vi "GSP_MasterConfiguration.vi"(5 "error in (no error)":errorcluster, 6 "Slit File":path, 7 "Filter File":path, 8 "grating file":path) -> (0 "error out":errorcluster, 2 "Changes Made?":bool)   [LabVIEW 2015]
uses:
  Misc/GUI_Buttons_23x22_W2K.llb/ArrowLeftBlue.ctl
  Misc/GUI_Buttons_23x22_W2K.llb/Delete1.ctl
  Dialog/dialog_messages.ctl
  GSP_GUI_global.vi
panel:
  in  "Clear Changes":bool
  in  "Load from Config":bool
  in  "Apply Changes":bool
  in  "Tab Control":T1(tab)=enum."Slit Carousel"
  in  "5-hole (SQUARE)":bool caption="6-hole (ROUND)"
  out "Filter Info":string
  in  "Remove Secondary":T2
  in  "Load Secondary":T3
  in  "Remove Primary":T2
  in  "Load Primary":T3
  in  "Available Filters":i32(listbox)
  in  "Secondary Filter Wheel Listbox":i32(listbox) caption="Secondary"
  in  "Primary Filter Wheel Listbox":i32(listbox) caption="Primary"
  out "Grating Info":string
  in  "Available Gratings":i32(listbox)
  in  "Remove  Grating":T2
  in  "Load Grating":T3
  in  "Grating Tray Listbox":i32(listbox)
  out "Slit Info":string
  in  "Available Slits":i32(listbox)
  in  "Remove  Slit":T2
  in  "Load Slit":T3
  in  "Slit Mask Listbox":i32(listbox)
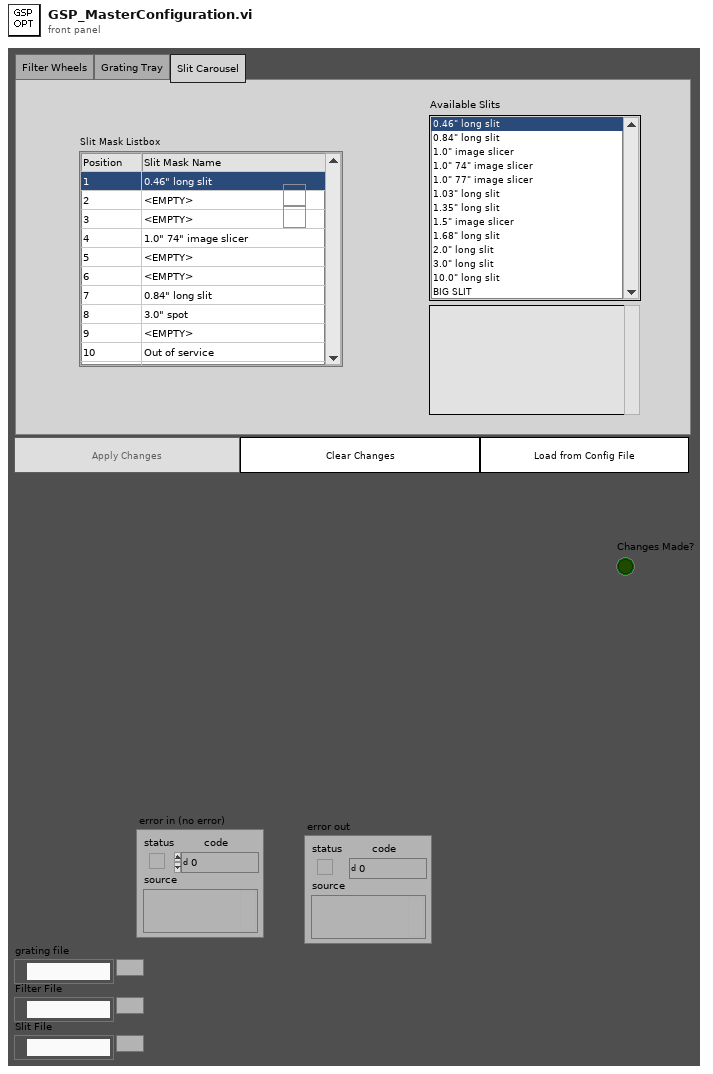
[diagram p1: front panel]
types:
  T1 = enum32{"Filter Wheels", "Grating Tray", "Slit Carousel"}
  T2 = typedef "Delete1.ctl" = bool
  T3 = typedef "ArrowLeftBlue.ctl" = bool
  T4 = typedef "dialog_messages.ctl" = enum16{"Custom", "Incompatible Config"}
  T5 = cluster{"Primary Filter Names":string[], "Secondary Filter Names":string[], "Grating Names":string[], "Slit Mask Names":string[]}
  T6 = cluster{"Comment":string, "lines/mm":i32, "modulation":dbl, "thickness (mm)":dbl}
  T7 = cluster{"Comment":string, "Width":dbl, "Observer":string, "Field":string}
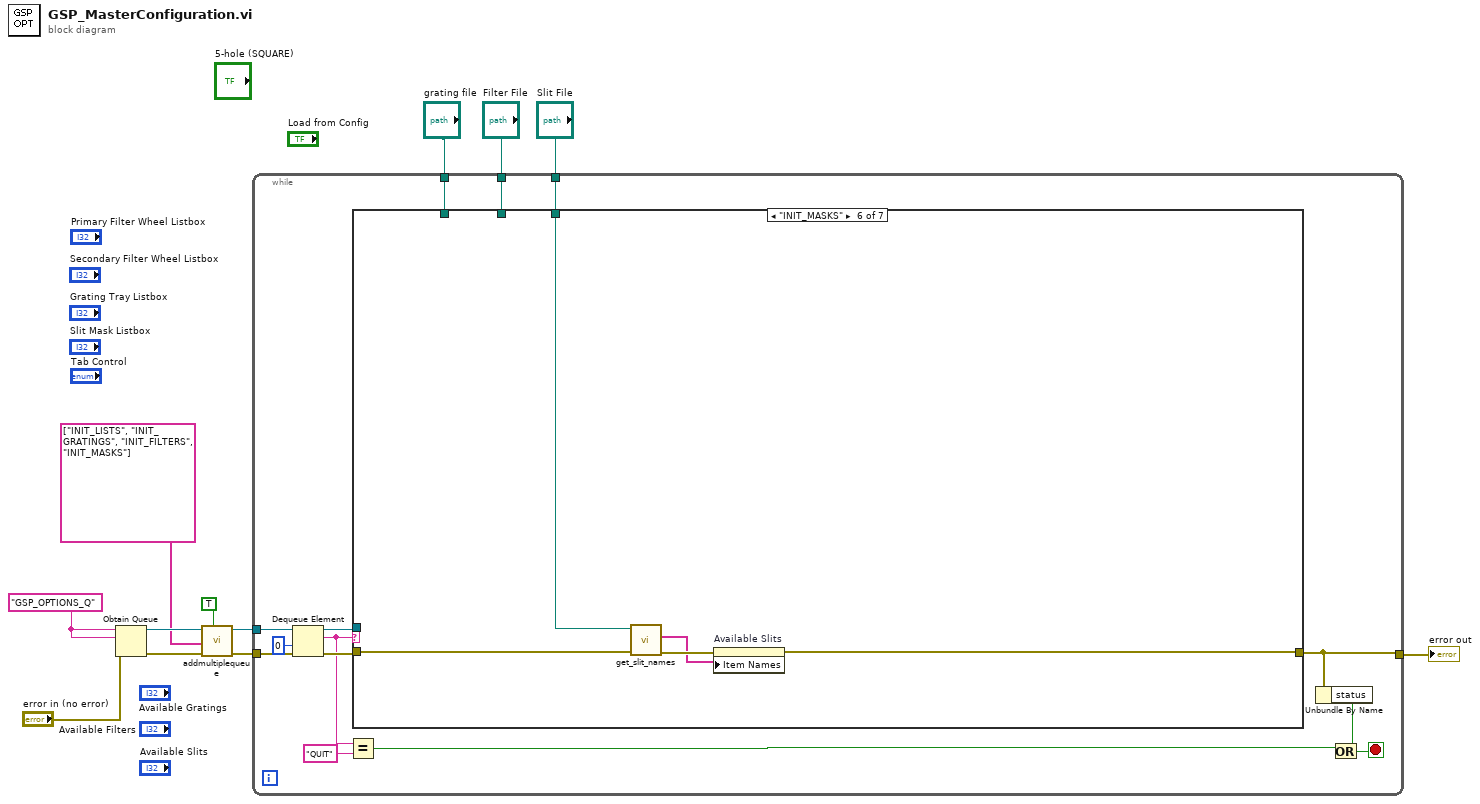
[diagram p0: block diagram]
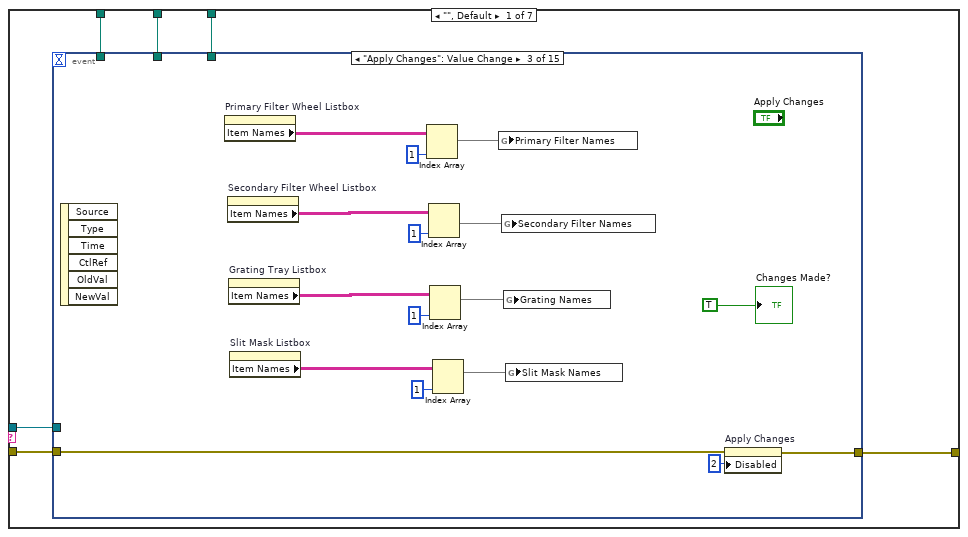
[diagram p2: hidden frame]
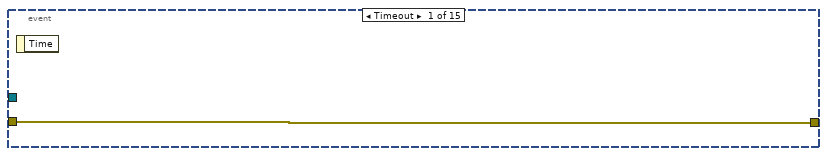
[diagram p3: hidden frame]
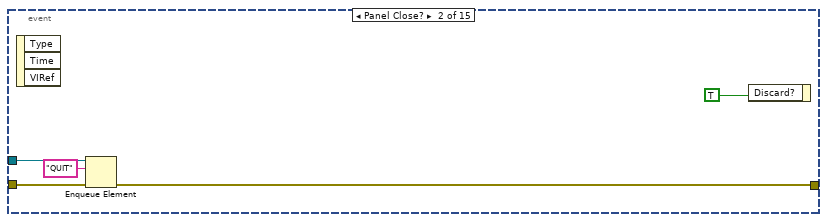
[diagram p4: hidden frame]
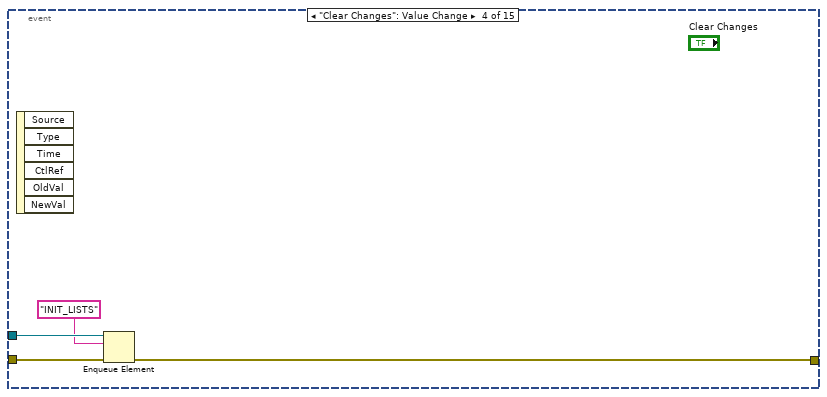
[diagram p5: hidden frame]
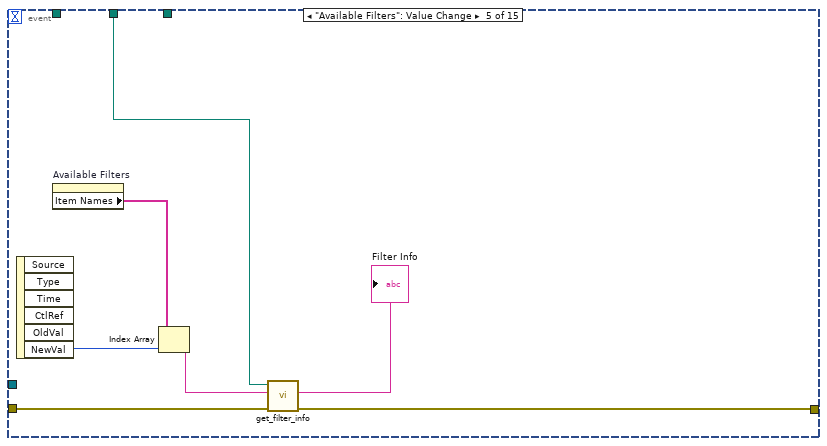
[diagram p6: hidden frame]
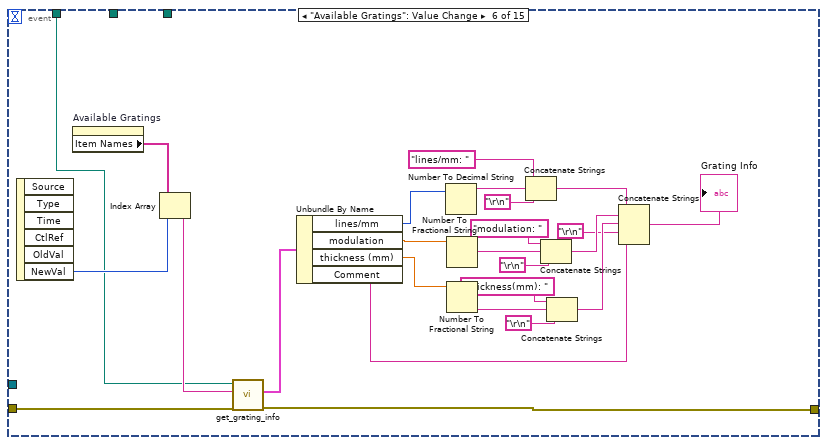
[diagram p7: hidden frame]
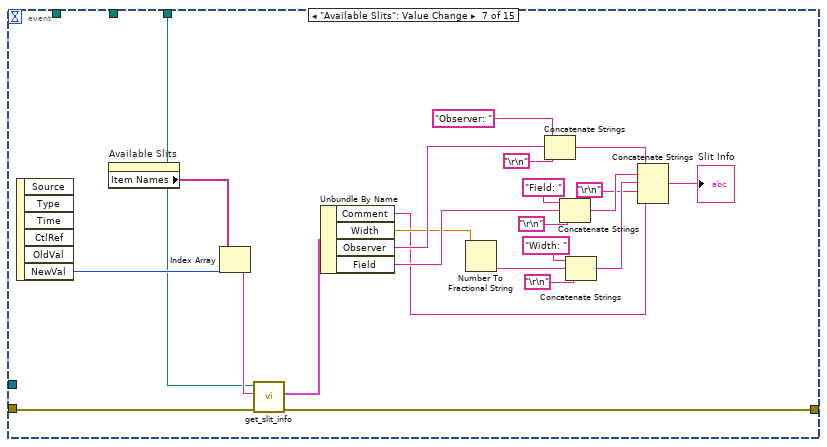
[diagram p8: hidden frame]
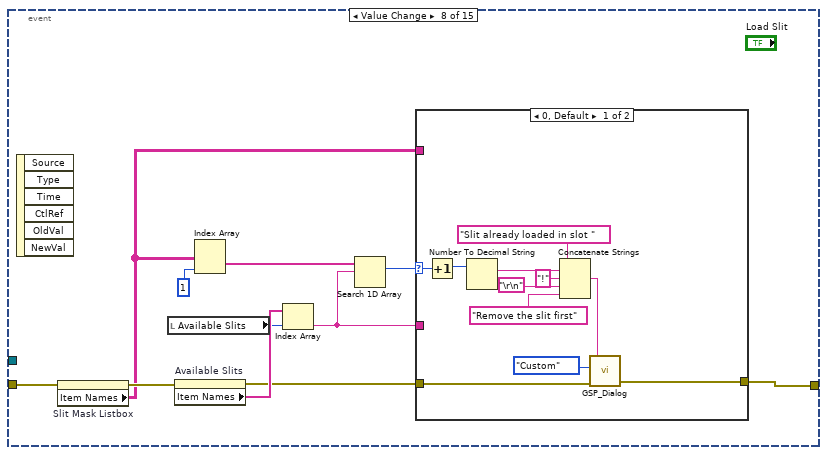
[diagram p9: hidden frame]
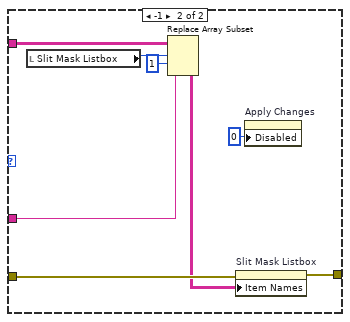
[diagram p10: hidden frame]
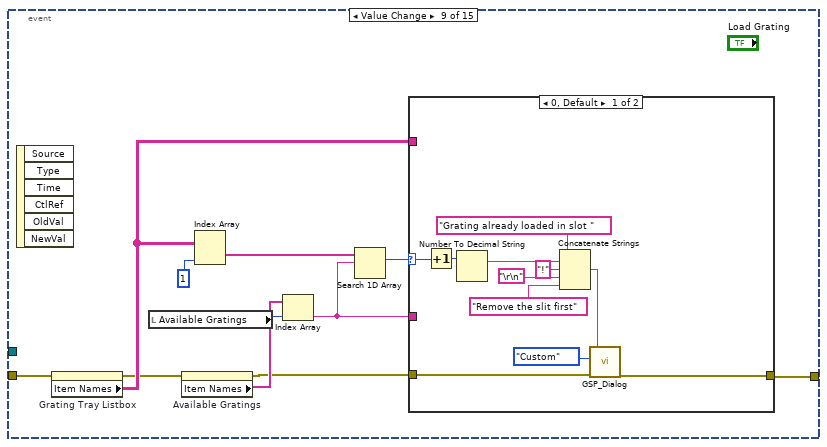
[diagram p11: hidden frame]
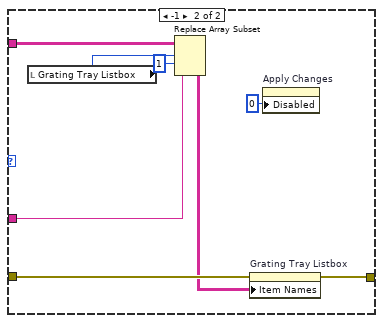
[diagram p12: hidden frame]
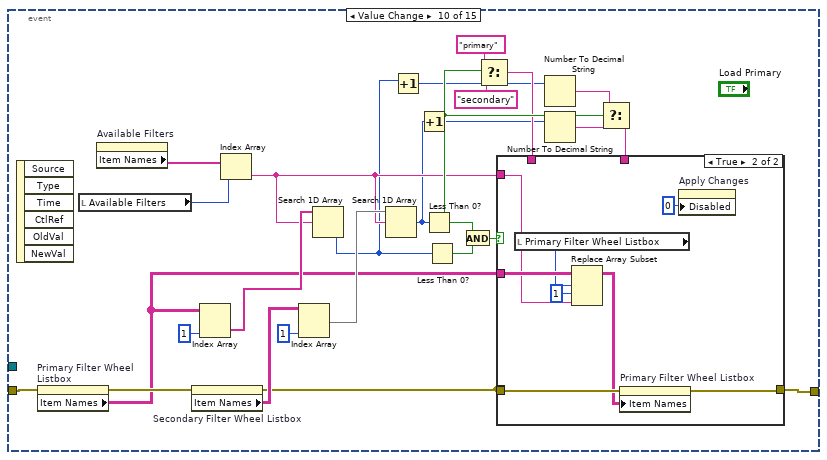
[diagram p13: hidden frame]
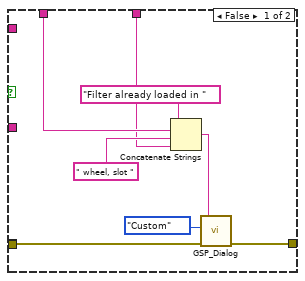
[diagram p14: hidden frame]
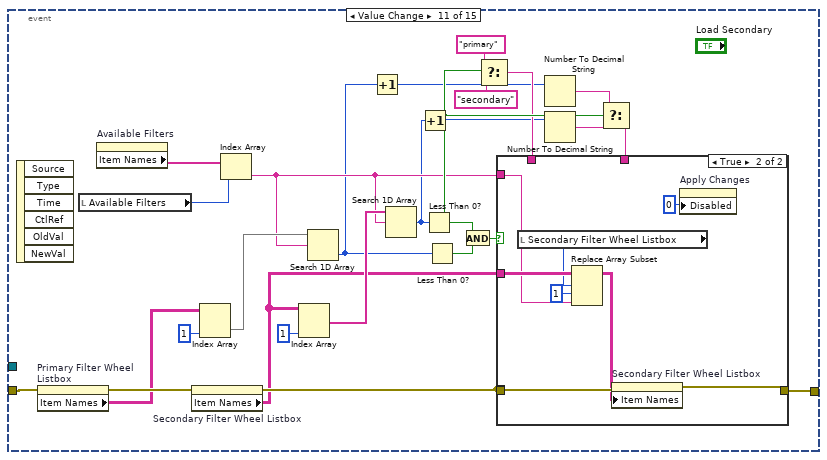
[diagram p15: hidden frame]
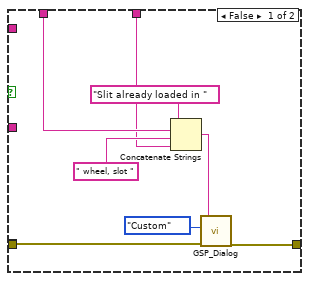
[diagram p16: hidden frame]
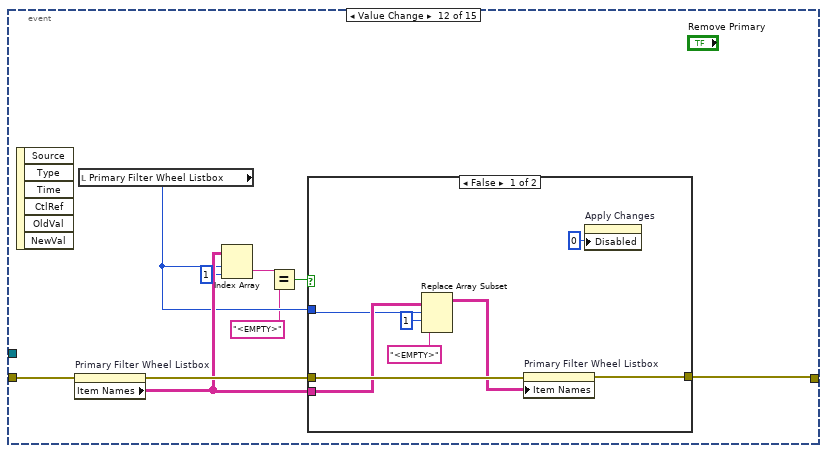
[diagram p17: hidden frame]
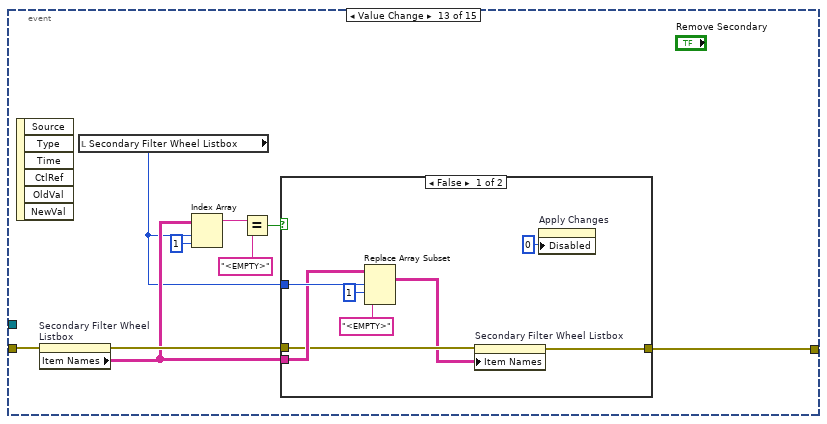
[diagram p19: hidden frame]
diagram:
  w12 = "GSP_OPTIONS_Q" ("name (unnamed)")
  n1 = Obtain Queue(name (unnamed)=w12, element data type=w12, error in (no error)="error in (no error)") -> (queue out=w11:refnum<queue>, error out=w10:errorcluster)  [unwired: 2 in, 1 out]
  n2 = call "addmultiplequeue.vi"("Add All (false)"=TRUE, "error in (no error)"=w10, "Strings to Add"=string[] ["INIT_LISTS", "INIT_GRATINGS", "INIT_FILTERS", "INIT_MASKS"], "queue"=w11) -> ("error out"=w9:errorcluster, "queue out"=w8:refnum<queue>)  [unwired: 3 in]
  n3 = while {
    tunnel: w9 -> [w25]
    tunnel: w8 -> [w26]
    tunnel: [w16] -> w6
    tunnel: "grating file" -> [w15]
    tunnel: "Filter File" -> [w14]
    tunnel: "Slit File" -> [w13]
    stop <- w19 stop-if-true
    n4 = Dequeue Element(queue=w26, timeout in ms (-1)=0, error in (no error)=w25) -> (queue out=w23:refnum<queue>, element=w21:string, error out=w22:errorcluster)  [unwired: 1 out]
    n5 = Equal?(x=w21, y="QUIT") -> (x = y?=w18:bool)
    n6 = case shown="\"INIT_MASKS\"" w21 {
      tunnel: w23 -> [w31 _ _ _ _ _ _]
      tunnel: w22 -> [w32 w345 w360 w384 w391 w396 w397]
      tunnel: [w30 w339 w360 w386 w388 w393 w397] -> w16
      tunnel: w15 -> [w28 _ _ w382 _ _ _]
      tunnel: w14 -> [w29 _ _ _ w387 _ _]
      tunnel: w13 -> [w27 _ _ _ _ w392 _]
      frame "", Default {
        n7 = event shown="[2] \"Apply Changes\": Value Change" {
          selector: _ -> [_ _ _ _ _ _ _ _ _ _ _ _ _ _ _]
          dyn-events: _ -> [_ _ _ _ _ _ _ _ _ _ _ _ _ _ _]
          timeout: _ -> [_ _ _ _ _ _ _ _ _ _ _ _ _ _ _]
          tunnel: w32 -> [w33 w36 w43 w57 w63 w68 w101 w124 w149 w199 w241 w266 w284 w302 w320]
          tunnel: w31 -> [_ w37 _ w58 _ _ _ _ _ _ _ _ _ _ _]
          tunnel: [w33 w35 w44 w56 w60 w69 w99 w117 w152 w188 w231 w264 w282 w300 w318] -> w30
          tunnel: w29 -> [_ _ _ _ w59 _ _ _ _ _ _ _ _ _ _]
          tunnel: w28 -> [_ _ _ _ _ w66 _ _ _ _ _ _ _ _ _]
          tunnel: w27 -> [_ _ _ _ _ _ w91 _ _ _ _ _ _ _ _]
          event Timeout {
            n8 = event-data() -> ()  [unwired: 1 in, 1 out]
          }
          event Panel Close? {
            n9 = event-data() -> ()  [unwired: 1 in, 3 out]
            n10 = Enqueue Element(queue=w37, element="QUIT", error in (no error)=w36) -> (error out=w35:errorcluster)  [unwired: 1 in, 2 out]
            n11 = event-data("Discard?"=TRUE) -> ()  [unwired: 1 in, 1 out]
          }
          event "Apply Changes": Value Change {
            n12 = event-data() -> ()  [unwired: 1 in, 6 out]
            n13 = property on="Primary Filter Wheel Listbox" class="MCListbox (strict)"() -> ("Item Names"=w53:string[][])  [unwired: 2 in, 2 out]
            n14 = property on="Secondary Filter Wheel Listbox" class="MCListbox (strict)"() -> ("Item Names"=w48:string[][])  [unwired: 2 in, 2 out]
            n15 = property on="Grating Tray Listbox" class="MCListbox (strict)"() -> ("Item Names"=w47:string[][])  [unwired: 2 in, 2 out]
            n16 = property on="Slit Mask Listbox" class="MCListbox (strict)"() -> ("Item Names"=w46:string[][])  [unwired: 2 in, 2 out]
            n17 = Index Array(array=w53, index (col)=1 ("disabled index (col)")) -> (element=w39:string[])  [unwired: 1 in]
            n18 = Index Array(array=w48, index (col)=1 ("disabled index (col)")) -> (element=w40:string[])  [unwired: 1 in]
            n19 = Index Array(array=w47, index (col)=1 ("disabled index (col)")) -> (element=w41:string[])  [unwired: 1 in]
            n20 = Index Array(array=w46, index (col)=1 ("disabled index (col)")) -> (element=w42:string[])  [unwired: 1 in]
            n21 = global write "GSP_GUI_global.vi" "Primary Filter Names"(w39) -> ()
            n22 = global write "GSP_GUI_global.vi" "Secondary Filter Names"(w40) -> ()
            n23 = global write "GSP_GUI_global.vi" "Grating Names"(w41) -> ()
            n24 = global write "GSP_GUI_global.vi" "Slit Mask Names"(w42) -> ()
            n25 = property on="Apply Changes" class="Bool"(error in=w43, "Disabled"=u8 2) -> (error out=w44:errorcluster)  [unwired: 1 in, 1 out]
            "Changes Made?" <- TRUE
          }
          event "Clear Changes": Value Change {
            n26 = event-data() -> ()  [unwired: 1 in, 6 out]
            n27 = Enqueue Element(queue=w58, element="INIT_LISTS", error in (no error)=w57) -> (error out=w56:errorcluster)  [unwired: 1 in, 2 out]
          }
          event "Available Filters": Value Change {
            n28 = event-data() -> ("NewVal"=w65:i32)  [unwired: 1 in, 5 out]
            n29 = property on="Available Filters" class="LstBox (strict)"() -> ("Item Names"=w64:string[])  [unwired: 2 in, 2 out]
            n30 = Index Array(array=w64, index=w65) -> (element=w62:string)
            n31 = call "get_filter_info.vi"("error in (no error)"=w63, "filter name"=w62, "configuration file path"=w59) -> ("error out"=w60:errorcluster, "Comment"=→"Filter Info":string)  [unwired: 3 in]
          }
          event "Available Gratings": Value Change {
            n32 = event-data() -> ("NewVal"=w90:i32)  [unwired: 1 in, 5 out]
            n33 = property on="Available Gratings" class="LstBox (strict)"() -> ("Item Names"=w89:string[])  [unwired: 2 in, 2 out]
            n34 = Index Array(array=w89, index=w90) -> (element=w67:string)
            n35 = call "get_grating_info.vi"("error in (no error)"=w68, "grating name"=w67, "configuration file path"=w66) -> ("error out"=w69:errorcluster, "Grating Info"=w70:T6)  [unwired: 3 in]
            n36 = Unbundle By Name(w70) -> ("lines/mm"=w88:i32, "modulation"=w87:dbl, "thickness (mm)"=w86:dbl, "Comment"=w73:string)
            n37 = Number To Decimal String(number=w88) -> (decimal integer string=w85:string)  [unwired: 1 in]
            n38 = Number To Fractional String(number=w87) -> (F-format string=w81:string)  [unwired: 3 in]
            n39 = Number To Fractional String(number=w86) -> (F-format string=w71:string)  [unwired: 3 in]
            n40 = Concatenate Strings("lines/mm: ", w85, "\r\n") -> (w77:string)
            n41 = Concatenate Strings("modulation: " ("string"), w81, "\r\n") -> (w76:string)
            n42 = Concatenate Strings("thickness(mm): " ("string"), w71, "\r\n") -> (w75:string)
            n43 = Concatenate Strings(w77, w76, w75, "\r\n", w73) -> (→"Grating Info":string)
          }
          event "Available Slits": Value Change {
            n44 = event-data() -> ("NewVal"=w113:i32)  [unwired: 1 in, 5 out]
            n45 = property on="Available Slits" class="LstBox (strict)"() -> ("Item Names"=w112:string[])  [unwired: 2 in, 2 out]
            n46 = Index Array(array=w112, index=w113) -> (element=w100:string)
            n47 = call "get_slit_info.vi"("error in (no error)"=w101, "mask name"=w100, "configuration file path"=w91) -> ("error out"=w99:errorcluster, "Slit Info"=w98:T7)  [unwired: 3 in]
            n48 = Unbundle By Name(w98) -> ("Comment"=w93:string, "Width"=w95:dbl, "Observer"=w97:string, "Field"=w96:string)
            n49 = Number To Fractional String(number=w95) -> (F-format string=w102:string)  [unwired: 3 in]
            n50 = Concatenate Strings("Observer: ", w97, "\r\n") -> (w94:string)
            n51 = Concatenate Strings("Field: " ("string"), w96, "\r\n") -> (w105:string)
            n52 = Concatenate Strings("Width: " ("string"), w102, "\r\n") -> (w104:string)
            n53 = Concatenate Strings(w94, w105, w104, "\r\n", w93) -> (→"Slit Info":string)
          }
          event Value Change {
            n54 = event-data() -> ()  [unwired: 1 in, 6 out]
            n55 = property on="Slit Mask Listbox" class="MCListbox (strict)"(error in=w124) -> (error out=w123:errorcluster, "Item Names"=w115:string[][])  [unwired: 1 in, 1 out]
            n56 = local read "Available Slits"() -> (w121:i32)
            n57 = property on="Available Slits" class="LstBox (strict)"(error in=w123) -> (error out=w118:errorcluster, "Item Names"=w122:string[])  [unwired: 1 in, 1 out]
            n58 = Index Array(array=w115, index (col)=1 ("disabled index (col)")) -> (element=w116:string[])  [unwired: 1 in]
            n59 = Index Array(array=w122, index=w121) -> (element=w114:string)
            n60 = Search 1D Array(1D array=w116, element=w114) -> (index of element=w119:i32)  [unwired: 1 in]
            n61 = case shown="0, Default" w119 {
              selector: w119 -> [w126 _]
              tunnel: w118 -> [w134 w143]
              tunnel: [w133 w142] -> w117
              tunnel: w115 -> [_ w141]
              tunnel: w114 -> [_ w138]
              frame 0, Default {
                n62 = Increment(x=w126) -> (x+1=w125:i32)
                n63 = Number To Decimal String(number=w125) -> (decimal integer string=w132:string)  [unwired: 1 in]
                n64 = Concatenate Strings("Slit already loaded in slot " ("Message"), w132, "!" ("string"), "\r\n", "Remove the slit first" ("string")) -> (w130:string)
                n65 = call "GSP_Dialog.vi"("error in (no error)"=w134, "Messages"=dialog_messages."Custom", "Message"=w130) -> ("error out"=w133:errorcluster)  [unwired: 4 in]
              }
              frame -1 {
                n66 = local read "Slit Mask Listbox"() -> (w139:i32)
                n67 = Replace Array Subset(array=w141, new element=w138, index (row)=w139, index (col)=1 ("disabled index (col)")) -> (w137:string[][])
                n68 = property on="Slit Mask Listbox" class="MCListbox (strict)"(error in=w143, "Item Names"=w137) -> (error out=w142:errorcluster)  [unwired: 1 in, 1 out]
                n69 = property on="Apply Changes" class="Bool"("Disabled"=u8 0) -> ()  [unwired: 2 in, 2 out]
              }
            }
          }
          event Value Change {
            n70 = event-data() -> ()  [unwired: 1 in, 6 out]
            n71 = property on="Grating Tray Listbox" class="MCListbox (strict)"(error in=w149) -> (error out=w147:errorcluster, "Item Names"=w148:string[][])  [unwired: 1 in, 1 out]
            n72 = local read "Available Gratings"() -> (w144:i32)
            n73 = property on="Available Gratings" class="LstBox (strict)"(error in=w147) -> (error out=w145:errorcluster, "Item Names"=w146:string[])  [unwired: 1 in, 1 out]
            n74 = Index Array(array=w148, index (col)=1 ("disabled index (col)")) -> (element=w151:string[])  [unwired: 1 in]
            n75 = Index Array(array=w146, index=w144) -> (element=w150:string)
            n76 = Search 1D Array(1D array=w151, element=w150) -> (index of element=w153:i32)  [unwired: 1 in]
            n77 = case shown="0, Default" w153 {
              selector: w153 -> [w156 _]
              tunnel: w145 -> [w164 w169]
              tunnel: [w163 w168] -> w152
              tunnel: w148 -> [_ w173]
              tunnel: w150 -> [_ w171]
              frame 0, Default {
                n78 = Increment(x=w156) -> (x+1=w155:i32)
                n79 = Number To Decimal String(number=w155) -> (decimal integer string=w162:string)  [unwired: 1 in]
                n80 = Concatenate Strings("Grating already loaded in slot " ("Message"), w162, "!" ("string"), "\r\n", "Remove the slit first" ("string")) -> (w160:string)
                n81 = call "GSP_Dialog.vi"("error in (no error)"=w164, "Messages"=dialog_messages."Custom", "Message"=w160) -> ("error out"=w163:errorcluster)  [unwired: 4 in]
              }
              frame -1 {
                n82 = local read "Grating Tray Listbox"() -> (w170:i32)
                n83 = Replace Array Subset(array=w173, new element=w171, index (row)=w170, index (col)=1 ("disabled index (col)")) -> (w167:string[][])
                n84 = property on="Grating Tray Listbox" class="MCListbox (strict)"(error in=w169, "Item Names"=w167) -> (error out=w168:errorcluster)  [unwired: 1 in, 1 out]
                n85 = property on="Apply Changes" class="Bool"("Disabled"=u8 0) -> ()  [unwired: 2 in, 2 out]
              }
            }
          }
          event Value Change {
            n86 = event-data() -> ()  [unwired: 1 in, 6 out]
            n87 = property on="Primary Filter Wheel Listbox" class="MCListbox (strict)"(error in=w199) -> (error out=w198:errorcluster, "Item Names"=w178:string[][])  [unwired: 1 in, 1 out]
            n88 = local read "Available Filters"() -> (w196:i32)
            n89 = property on="Available Filters" class="LstBox (strict)"() -> ("Item Names"=w197:string[])  [unwired: 2 in, 2 out]
            n90 = property on="Secondary Filter Wheel Listbox" class="MCListbox (strict)"(error in=w198) -> (error out=w179:errorcluster, "Item Names"=w193:string[][])  [unwired: 1 in, 1 out]
            n91 = Index Array(array=w178, index (col)=1 ("disabled index (col)")) -> (element=w192:string[])  [unwired: 1 in]
            n92 = Index Array(array=w197, index=w196) -> (element=w180:string)
            n93 = Index Array(array=w193, index (col)=1 ("disabled index (col)")) -> (element=w191:string[])  [unwired: 1 in]
            n94 = Search 1D Array(1D array=w192, element=w180) -> (index of element=w177:i32)  [unwired: 1 in]
            n95 = Search 1D Array(1D array=w191, element=w180) -> (index of element=w175:i32)  [unwired: 1 in]
            n96 = Increment(x=w177) -> (x+1=w176:i32)
            n97 = Increment(x=w175) -> (x+1=w174:i32)
            n98 = Less Than 0?(x=w175) -> (x < 0?=w183:bool)
            n99 = Less Than 0?(x=w177) -> (x < 0?=w190:bool)
            n100 = And(x=w183, y=w190) -> (x .and. y?=w189:bool)
            n101 = Select(t="primary", s=w183, f="secondary") -> (s? t:f=w182:string)
            n102 = Number To Decimal String(number=w176) -> (decimal integer string=w185:string)  [unwired: 1 in]
            n103 = Number To Decimal String(number=w174) -> (decimal integer string=w184:string)  [unwired: 1 in]
            n104 = Select(t=w185, s=w183, f=w184) -> (s? t:f=w181:string)
            n105 = case shown="True" w189 {
              tunnel: w179 -> [w205 _]
              tunnel: [w204 w214] -> w188
              tunnel: w182 -> [w202 _]
              tunnel: w181 -> [w200 _]
              tunnel: w180 -> [_ w210]
              tunnel: w179 -> [_ w215]
              tunnel: w178 -> [_ w213]
              frame False {
                n106 = Concatenate Strings("Filter already loaded in " ("Message"), w202, " wheel, slot ", w200) -> (w206:string)
                n107 = call "GSP_Dialog.vi"("error in (no error)"=w205, "Messages"=dialog_messages."Custom", "Message"=w206) -> ("error out"=w204:errorcluster)  [unwired: 4 in]
              }
              frame True {
                n108 = local read "Primary Filter Wheel Listbox"() -> (w211:i32)
                n109 = Replace Array Subset(array=w213, new element=w210, index (row)=w211, index (col)=1 ("disabled index (col)")) -> (w209:string[][])
                n110 = property on="Primary Filter Wheel Listbox" class="MCListbox (strict)"(error in=w215, "Item Names"=w209) -> (error out=w214:errorcluster)  [unwired: 1 in, 1 out]
                n111 = property on="Apply Changes" class="Bool"("Disabled"=u8 0) -> ()  [unwired: 2 in, 2 out]
              }
            }
          }
          event Value Change {
            n112 = event-data() -> ()  [unwired: 1 in, 6 out]
            n113 = property on="Primary Filter Wheel Listbox" class="MCListbox (strict)"(error in=w241) -> (error out=w240:errorcluster, "Item Names"=w223:string[][])  [unwired: 1 in, 1 out]
            n114 = local read "Available Filters"() -> (w238:i32)
            n115 = property on="Available Filters" class="LstBox (strict)"() -> ("Item Names"=w239:string[])  [unwired: 2 in, 2 out]
            n116 = property on="Secondary Filter Wheel Listbox" class="MCListbox (strict)"(error in=w240) -> (error out=w224:errorcluster, "Item Names"=w222:string[][])  [unwired: 1 in, 1 out]
            n117 = Index Array(array=w223, index (col)=1 ("disabled index (col)")) -> (element=w235:string[])  [unwired: 1 in]
            n118 = Index Array(array=w239, index=w238) -> (element=w225:string)
            n119 = Index Array(array=w222, index (col)=1 ("disabled index (col)")) -> (element=w234:string[])  [unwired: 1 in]
            n120 = Search 1D Array(1D array=w235, element=w225) -> (index of element=w219:i32)  [unwired: 1 in]
            n121 = Increment(x=w219) -> (x+1=w218:i32)
            n122 = Search 1D Array(1D array=w234, element=w225) -> (index of element=w217:i32)  [unwired: 1 in]
            n123 = Increment(x=w217) -> (x+1=w216:i32)
            n124 = Less Than 0?(x=w217) -> (x < 0?=w228:bool)
            n125 = Less Than 0?(x=w219) -> (x < 0?=w233:bool)
            n126 = And(x=w228, y=w233) -> (x .and. y?=w232:bool)
            n127 = Select(t="primary", s=w228, f="secondary") -> (s? t:f=w227:string)
            n128 = Number To Decimal String(number=w218) -> (decimal integer string=w220:string)  [unwired: 1 in]
            n129 = Number To Decimal String(number=w216) -> (decimal integer string=w221:string)  [unwired: 1 in]
            n130 = Select(t=w220, s=w228, f=w221) -> (s? t:f=w226:string)
            n131 = case shown="True" w232 {
              tunnel: w224 -> [w247 w253]
              tunnel: [w246 w251] -> w231
              tunnel: w227 -> [w244 _]
              tunnel: w226 -> [w242 _]
              tunnel: w225 -> [_ w255]
              tunnel: w224 -> [_ _]
              tunnel: w222 -> [_ w257]
              frame False {
                n132 = Concatenate Strings("Slit already loaded in " ("Message"), w244, " wheel, slot ", w242) -> (w248:string)
                n133 = call "GSP_Dialog.vi"("error in (no error)"=w247, "Messages"=dialog_messages."Custom", "Message"=w248) -> ("error out"=w246:errorcluster)  [unwired: 4 in]
              }
              frame True {
                n134 = local read "Secondary Filter Wheel Listbox"() -> (w254:i32)
                n135 = Replace Array Subset(array=w257, new element=w255, index (row)=w254, index (col)=1 ("disabled index (col)")) -> (w252:string[][])
                n136 = property on="Secondary Filter Wheel Listbox" class="MCListbox (strict)"(error in=w253, "Item Names"=w252) -> (error out=w251:errorcluster)  [unwired: 1 in, 1 out]
                n137 = property on="Apply Changes" class="Bool"("Disabled"=u8 0) -> ()  [unwired: 2 in, 2 out]
              }
            }
          }
          event Value Change {
            n138 = event-data() -> ()  [unwired: 1 in, 6 out]
            n139 = property on="Primary Filter Wheel Listbox" class="MCListbox (strict)"(error in=w266) -> (error out=w265:errorcluster, "Item Names"=w263:string[][])  [unwired: 1 in, 1 out]
            n140 = local read "Primary Filter Wheel Listbox"() -> (w261:i32)
            n141 = Index Array(array=w263, index (row)=w261, index (col)=1 ("disabled index (col)")) -> (element=w260:string)
            n142 = Equal?(x=w260, y="<EMPTY>") -> (x = y?=w258:bool)
            n143 = case shown="False" w258 {
              tunnel: w265 -> [w272 w275]
              tunnel: [w271 w275] -> w264
              tunnel: w263 -> [w269 _]
              tunnel: w261 -> [w268 _]
              frame False {
                n144 = Replace Array Subset(array=w269, new element="<EMPTY>" ("new element/subarray"), index (row)=w268, index (col)=1 ("disabled index (col)")) -> (w270:string[][])
                n145 = property on="Primary Filter Wheel Listbox" class="MCListbox (strict)"(error in=w272, "Item Names"=w270) -> (error out=w271:errorcluster)  [unwired: 1 in, 1 out]
                n146 = property on="Apply Changes" class="Bool"("Disabled"=u8 0) -> ()  [unwired: 2 in, 2 out]
              }
              frame True {
              }
            }
          }
          event Value Change {
            n147 = event-data() -> ()  [unwired: 1 in, 6 out]
            n148 = property on="Secondary Filter Wheel Listbox" class="MCListbox (strict)"(error in=w284) -> (error out=w283:errorcluster, "Item Names"=w281:string[][])  [unwired: 1 in, 1 out]
            n149 = local read "Secondary Filter Wheel Listbox"() -> (w279:i32)
            n150 = Index Array(array=w281, index (row)=w279, index (col)=1 ("disabled index (col)")) -> (element=w277:string)
            n151 = Equal?(x=w277, y="<EMPTY>" ("new element/subarray")) -> (x = y?=w278:bool)
            n152 = case shown="False" w278 {
              tunnel: w279 -> [w291 _]
              tunnel: w281 -> [w290 _]
              tunnel: w283 -> [w289 w293]
              tunnel: [w287 w293] -> w282
              frame False {
                n153 = Replace Array Subset(array=w290, new element="<EMPTY>" ("new element/subarray"), index (row)=w291, index (col)=1 ("disabled index (col)")) -> (w288:string[][])
                n154 = property on="Secondary Filter Wheel Listbox" class="MCListbox (strict)"(error in=w289, "Item Names"=w288) -> (error out=w287:errorcluster)  [unwired: 1 in, 1 out]
                n155 = property on="Apply Changes" class="Bool"("Disabled"=u8 0) -> ()  [unwired: 2 in, 2 out]
              }
              frame True {
              }
            }
          }
          event Value Change {
            n156 = event-data() -> ()  [unwired: 1 in, 6 out]
            n157 = property on="Slit Mask Listbox" class="MCListbox (strict)"(error in=w302) -> (error out=w301:errorcluster, "Item Names"=w299:string[][])  [unwired: 1 in, 1 out]
            n158 = local read "Slit Mask Listbox"() -> (w297:i32)
            n159 = Index Array(array=w299, index (row)=w297, index (col)=1 ("disabled index (col)")) -> (element=w295:string)
            n160 = Equal?(x=w295, y="<EMPTY>" ("new element/subarray")) -> (x = y?=w296:bool)
            n161 = case shown="False" w296 {
              tunnel: w301 -> [w310 w311]
              tunnel: w299 -> [w309 _]
              tunnel: w297 -> [w307 _]
              tunnel: [w305 w311] -> w300
              frame False {
                n162 = Replace Array Subset(array=w309, new element="<EMPTY>" ("new element/subarray"), index (row)=w307, index (col)=1 ("disabled index (col)")) -> (w306:string[][])
                n163 = property on="Slit Mask Listbox" class="MCListbox (strict)"(error in=w310, "Item Names"=w306) -> (error out=w305:errorcluster)  [unwired: 1 in, 1 out]
                n164 = property on="Apply Changes" class="Bool"("Disabled"=u8 0) -> ()  [unwired: 2 in, 2 out]
              }
              frame True {
              }
            }
          }
          event Value Change {
            n165 = event-data() -> ()  [unwired: 1 in, 6 out]
            n166 = property on="Grating Tray Listbox" class="MCListbox (strict)"(error in=w320) -> (error out=w319:errorcluster, "Item Names"=w317:string[][])  [unwired: 1 in, 1 out]
            n167 = local read "Grating Tray Listbox"() -> (w315:i32)
            n168 = Index Array(array=w317, index (row)=w315, index (col)=1 ("disabled index (col)")) -> (element=w313:string)
            n169 = Equal?(x=w313, y="<EMPTY>" ("new element/subarray")) -> (x = y?=w314:bool)
            n170 = case shown="False" w314 {
              tunnel: w315 -> [w327 _]
              tunnel: w317 -> [w326 _]
              tunnel: w319 -> [w325 w329]
              tunnel: [w323 w329] -> w318
              frame False {
                n171 = Replace Array Subset(array=w326, new element="<EMPTY>" ("new element/subarray"), index (row)=w327, index (col)=1 ("disabled index (col)")) -> (w324:string[][])
                n172 = property on="Grating Tray Listbox" class="MCListbox (strict)"(error in=w325, "Item Names"=w324) -> (error out=w323:errorcluster)  [unwired: 1 in, 1 out]
                n173 = property on="Apply Changes" class="Bool"("Disabled"=u8 0) -> ()  [unwired: 2 in, 2 out]
              }
              frame True {
              }
            }
          }
        }
      }
      frame "UPDATE_GRATING_MASK" {
        n174 = property on="Slit Mask Listbox" class="MCListbox (strict)"(error in=w345) -> (error out=w332:errorcluster, "Item Names"=w344:string[][])  [unwired: 1 in, 1 out]
        n175 = Index Array(array=w344, index (col)=1 ("disabled index (col)")) -> (element=w341:string[])  [unwired: 1 in]
        n176 = global write "GSP_GUI_global.vi" "Slit Mask Names"(w341) -> ()
        n177 = property on="Grating Tray Listbox" class="MCListbox (strict)"(error in=w332) -> (error out=w331:errorcluster, "Item Names"=w342:string[][])  [unwired: 1 in, 1 out]
        n178 = Index Array(array=w342, index (col)=1 ("disabled index (col)")) -> (element=w340:string[])  [unwired: 1 in]
        n179 = global write "GSP_GUI_global.vi" "Grating Names"(w340) -> ()
        n180 = stacked-sequence {
          tunnel: [w350] -> w337
          tunnel: [w349] -> w336
          tunnel: [w348] -> w335
          tunnel: [w347] -> w334
          tunnel: w331 -> [_]
          frame #0 {
            n181 = global read "GSP_GUI_global.vi" "Secondary Filter Names"() -> (w350:string[])
            n182 = global read "GSP_GUI_global.vi" "Primary Filter Names"() -> (w347:string[])
            n183 = global read "GSP_GUI_global.vi" "Slit Mask Names"() -> (w348:string[])
            n184 = global read "GSP_GUI_global.vi" "Grating Names"() -> (w349:string[])
          }
        }
        n185 = global read "GSP_GUI_global.vi" "Configuration File"() -> (w330:path)
        n186 = Bundle By Name(cluster=T5 {"Primary Filter Names"=[], "Secondary Filter Names"=[], "Grating Names"=[], "Slit Mask Names"=[]} ("Present Configuration"), "Primary Filter Names"=w334, "Secondary Filter Names"=w337, "Grating Names"=w336, "Slit Mask Names"=w335) -> (w333:T5)
        n187 = call "Write_Master_Config.vi"("error in (no error)"=w331, "Present Configuration"=w333, "configuration file path"=w330) -> ("error out"=w339:errorcluster)  [unwired: 4 in]
      }
      frame "INIT_LISTS" {
        w352 = 0
        n188 = global read "GSP_GUI_global.vi" "Slit Mask Names"() -> (w361:string[])
        n189 = for {
          tunnel: w361 -> [w380] mode=indexing
          tunnel: [w379] -> w359 mode=indexing
          i -> [w378]
          n190 = Increment(x=w378) -> (x+1=w377:i32)
          n191 = Number To Decimal String(number=w377) -> (decimal integer string=w381:string)  [unwired: 1 in]
          n192 = Build Array(w381, w380) -> (w379:string[])
        }
        n193 = global read "GSP_GUI_global.vi" "Primary Filter Names"() -> (w357:string[])
        n194 = for {
          tunnel: w357 -> [w370] mode=indexing
          tunnel: [w369] -> w354 mode=indexing
          i -> [w368]
          n195 = Increment(x=w368) -> (x+1=w367:i32)
          n196 = Number To Decimal String(number=w367) -> (decimal integer string=w371:string)  [unwired: 1 in]
          n197 = Build Array(w371, w370) -> (w369:string[])
        }
        n198 = property on="Primary Filter Wheel Listbox" class="MCListbox (strict)"("Item Names"=w354) -> ()  [unwired: 2 in, 2 out]
        n199 = property on="Slit Mask Listbox" class="MCListbox (strict)"("Item Names"=w359) -> ()  [unwired: 2 in, 2 out]
        n200 = local write "Primary Filter Wheel Listbox"(w352) -> ()
        n201 = local write "Secondary Filter Wheel Listbox"(w352) -> ()
        n202 = local write "Slit Mask Listbox"(w352) -> ()
        n203 = local write "Grating Tray Listbox"(w352) -> ()
        n204 = global read "GSP_GUI_global.vi" "Grating Names"() -> (w358:string[])
        n205 = for {
          tunnel: w358 -> [w375] mode=indexing
          tunnel: [w374] -> w355 mode=indexing
          i -> [w373]
          n206 = Increment(x=w373) -> (x+1=w372:i32)
          n207 = Number To Decimal String(number=w372) -> (decimal integer string=w376:string)  [unwired: 1 in]
          n208 = Build Array(w376, w375) -> (w374:string[])
        }
        n209 = global read "GSP_GUI_global.vi" "Secondary Filter Names"() -> (w356:string[])
        n210 = for {
          tunnel: w356 -> [w365] mode=indexing
          tunnel: [w364] -> w353 mode=indexing
          i -> [w363]
          n211 = Increment(x=w363) -> (x+1=w362:i32)
          n212 = Number To Decimal String(number=w362) -> (decimal integer string=w366:string)  [unwired: 1 in]
          n213 = Build Array(w366, w365) -> (w364:string[])
        }
        n214 = property on="Grating Tray Listbox" class="MCListbox (strict)"("Item Names"=w355) -> ()  [unwired: 2 in, 2 out]
        n215 = property on="Secondary Filter Wheel Listbox" class="MCListbox (strict)"("Item Names"=w353) -> ()  [unwired: 2 in, 2 out]
        n216 = property on="Apply Changes" class="Bool"("Disabled"=u8 2) -> ()  [unwired: 2 in, 2 out]
      }
      frame "INIT_GRATINGS" {
        n217 = call "get_grating_names.vi"("error in (no error)"=w384, "grating file"=w382) -> ("error out"=w385:errorcluster, "grating names"=w383:string[])  [unwired: 3 in, 1 out]
        n218 = property on="Available Gratings" class="LstBox (strict)"(error in=w385, "Item Names"=w383) -> (error out=w386:errorcluster)  [unwired: 1 in, 1 out]
      }
      frame "INIT_FILTERS" {
        n219 = call "get_filter_names.vi"("error in (no error)"=w391, "filter file"=w387) -> ("error out"=w390:errorcluster, "filter names"=w389:string[])  [unwired: 3 in, 1 out]
        n220 = property on="Available Filters" class="LstBox (strict)"(error in=w390, "Item Names"=w389) -> (error out=w388:errorcluster)  [unwired: 1 in, 1 out]
      }
      frame "INIT_MASKS" {
        n221 = call "get_slit_names.vi"("error in (no error)"=w396, "slit file"=w392) -> ("error out"=w395:errorcluster, "slit names"=w394:string[])  [unwired: 3 in, 1 out]
        n222 = property on="Available Slits" class="LstBox (strict)"(error in=w395, "Item Names"=w394) -> (error out=w393:errorcluster)  [unwired: 1 in, 1 out]
      }
      frame "QUIT" {
      }
    }
    n223 = Unbundle By Name(w16) -> ("status"=w17:bool)
    n224 = Or(x=w18, y=w17) -> (x .or. y?=w19:bool)
  }
  "error out" <- w6
